vi "I2C_Start.vi"(5 "TransmitDelay(Ticks)":u32, 7 "HalfCycle(Ticks)":u32, 8 "error in":errorcluster) -> (0 "error out":errorcluster)   [LabVIEW 2019]
doc: "Sends a START out the I2C Bus. \n\n<b>Inputs:</b>\n---------------------\n<b>HalfCycle(Ticks)</b> this the number of FPGA clock cycles in half og the clock period. Therefore twice this number yields the clock period, in ticks.\n\n<b>TransmitDelay(Ticks)</b> the delay in FPGA clock cycles before writing bytes on SDA.\n---------------------\nSee block diagram for more details on the implementation details.\n\nAuthor:\nPeter Fuller\nSenior Engineer\nPLF Consulting, LLC\n\nemail: peter@plfconsulting.com\nphone: 617.699.2201"
uses:
  <vilib>/eio/EIONode/EIONode.xnode
  Instance           5 17Saved   I2C_Start .vi
  Instance           1 17Saved   I2C_Start .vi
  <vilib>/eio/EIOMethodNode/EIOMethodNode.xnode
  Instance           2 17Saved   I2C_Start .vi
  <vilib>/rvi/eio/common/nirviEmuTemplateMethod_errors.vi
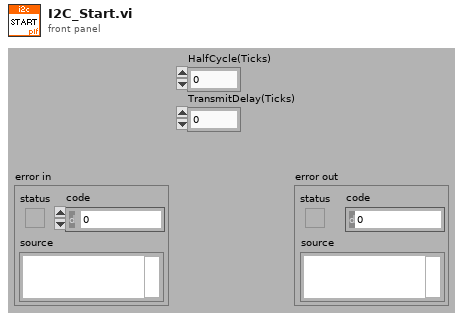
[diagram p1: front panel]
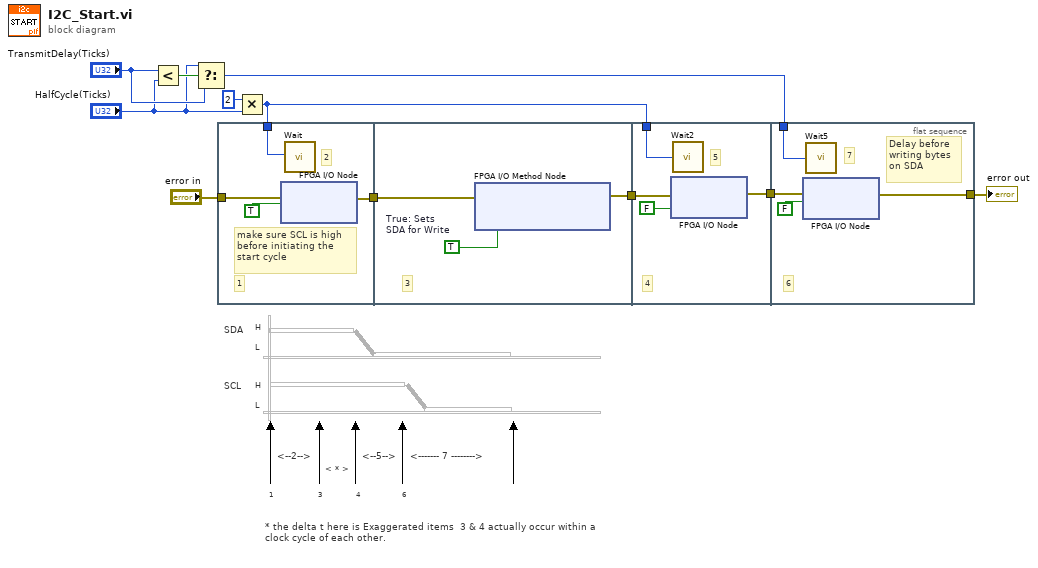
[diagram p0: block diagram]
diagram:
  # "6"
  # "H\n\nL"
  # "H\n\nL"
  # "* the delta t here is Exaggerated items  3 & 4 actually occur within a clock cycle of each other."
  # "< * >"
  # "4"
  # "<------- 7 -------->"
  # "<--5-->"
  # "<--2-->"
  # "3"
  # "1"
  # "SCL"
  # "SDA"
  n1 = Less?(x="TransmitDelay(Ticks)", y="HalfCycle(Ticks)") -> (x < y?=w10:bool)
  n2 = Select(t="HalfCycle(Ticks)", s=w10, f="TransmitDelay(Ticks)") -> (s? t:f=w1:u32)
  n3 = flat-sequence {
    tunnel: "error in" -> [w14]
    tunnel: [w13] -> w4
    tunnel: w3 -> [w12]
    tunnel: w4 -> [w17]
    tunnel: [w16] -> w5
    tunnel: [w21] -> w2
    tunnel: w5 -> [w20]
    tunnel: w3 -> [w19]
    tunnel: w2 -> [w25]
    tunnel: w1 -> [w23]
    tunnel: [w24] -> w11
    frame #0 {
      # "2"
      # "1"
      # "make sure SCL is high \nbefore initiating the\nstart cycle"
      n4 = xnode "FPGA I/O Node"("error in"=w14, "SCL"=TRUE ("Value")) -> ("error out"=w13:errorcluster)  [unwired: 1 in, 1 out]
      n5 = call "Wait"("Count(Ticks)"=w12) -> ()  [unwired: 1 out]
    }
    frame #1 {
      w18 = TRUE  # True: Sets  SDA for Write
      # "3"
      n6 = xnode "FPGA I/O Method Node"("error in"=w17, "Enable"=w18) -> ("error out"=w16:errorcluster)  [unwired: 1 in, 1 out]
    }
    frame #2 {
      # "5"
      # "4"
      n7 = xnode "FPGA I/O Node"("error in"=w20, "SDA"=FALSE ("Value")) -> ("error out"=w21:errorcluster)  [unwired: 1 in, 1 out]
      n8 = call "Wait2"("Count(Ticks)"=w19) -> ()  [unwired: 1 out]
    }
    frame #3 {
      # "7"
      # "Delay before\nwriting bytes \non SDA"
      # "6"
      n9 = xnode "FPGA I/O Node"("error in"=w25, "SCL"=FALSE ("Value")) -> ("error out"=w24:errorcluster)  [unwired: 1 in, 1 out]
      n10 = call "Wait5"("Count(Ticks)"=w23) -> ()  [unwired: 1 out]
    }
  }
  n11 = Multiply(x=u32 2, y="HalfCycle(Ticks)") -> (x*y=w3:u32)
  "error out" <- w11
